vi "Manual User Input.vi"() -> (2 "XML":path, 3 "ZIP":path, 4 "Cancelled?":bool=TRUE)   [LabVIEW 2021]
panel:
  in  "Loc string":string="LabVIEW cannot reach the National Instruments Web server. You must synchronize with the Icon Library manually.\nClick the Help button for more information about resolving this error."
  in  "Help":bool
  in  "Icon library XML file":path
  in  "Icon library ZIP file":path
  out "Instructions":string
  in  "Cancel":bool
  in  "OK":bool
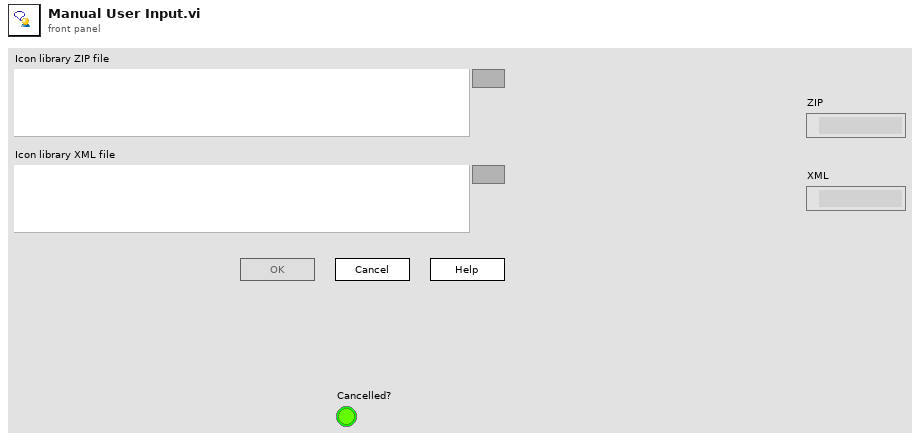
[diagram p1: front panel]
types:
  T1 = enum8{"Enabled", "Disabled", "Disabled and Grayed Out"}
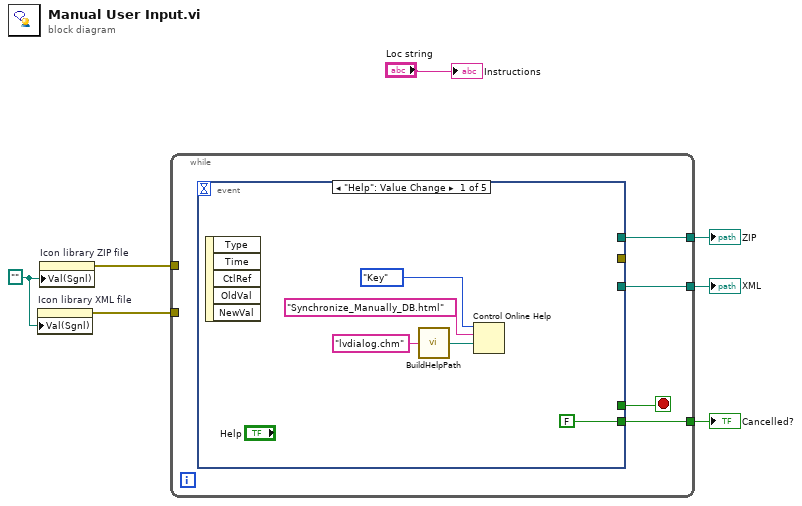
[diagram p0: block diagram]
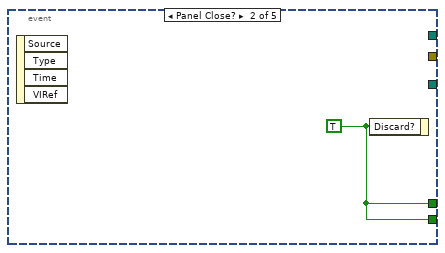
[diagram p2: hidden frame]
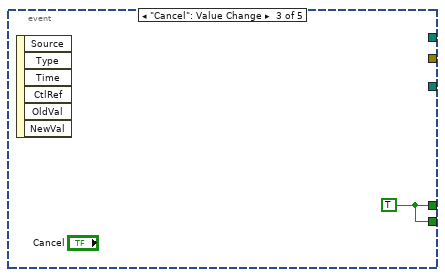
[diagram p3: hidden frame]
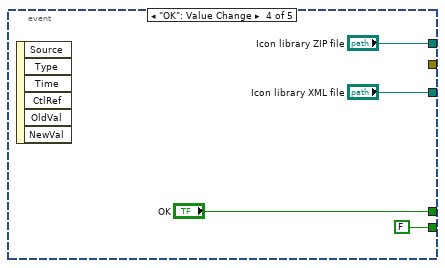
[diagram p4: hidden frame]
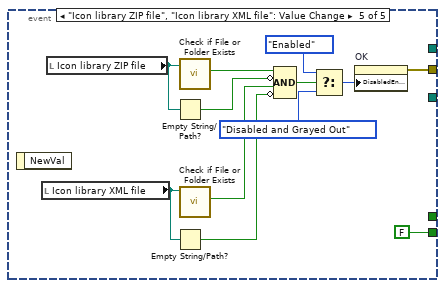
[diagram p5: hidden frame]
diagram:
  w5 = path ""
  n1 = property on="Icon library XML file" class="Path"("Val(Sgnl)"=w5) -> (error out=w2:errorcluster)  [unwired: 2 in, 1 out]
  n2 = property on="Icon library ZIP file" class="Path"("Val(Sgnl)"=w5) -> (error out=w3:errorcluster)  [unwired: 2 in, 1 out]
  n3 = while {
    tunnel: [w8] -> w7
    tunnel: [w11] -> w4
    tunnel: [w10] -> w6
    tunnel: w3 -> [_]
    tunnel: w2 -> [_]
    stop <- w9 stop-if-true
    n4 = event shown="[0] \"Help\": Value Change" {
      selector: _ -> [_ _ _ _ _]
      dyn-events: _ -> [_ _ _ _ _]
      timeout: _ -> [_ _ _ _ _]
      tunnel: [_ w17 w18 "OK" _] -> w9
      tunnel: [_ _ _ "Icon library ZIP file" _] -> w11
      tunnel: [_ _ _ "Icon library XML file" _] -> w10
      tunnel: [_ _ _ _ w24] -> _
      tunnel: [FALSE ("Discard?") w17 w18 FALSE ("Discard?") FALSE ("Discard?")] -> w8
      event "Help": Value Change {
        n5 = event-data() -> ()  [unwired: 1 in, 5 out]
        n6 = call <vilib>:"BuildHelpPath.vi"("Help File Name"="lvdialog.chm") -> ("Help File Path"=w14:path)
        n7 = Control Online Help(2:w14, 3:"Synchronize_Manually_DB.html" ("String to search for"), 4:enum16{"Contents", "Key", "Close"}."Key" ("Operation")) -> ()  [unwired: 1 in, 1 out]
      }
      event Panel Close? {
        w17 = TRUE ("Discard?")
        n8 = event-data() -> ()  [unwired: 1 in, 4 out]
        n9 = event-data("Discard?"=w17) -> ()  [unwired: 1 in, 1 out]
      }
      event "Cancel": Value Change {
        w18 = TRUE ("Discard?")
        n10 = event-data() -> ()  [unwired: 1 in, 6 out]
      }
      event "OK": Value Change {
        n11 = event-data() -> ()  [unwired: 1 in, 6 out]
      }
      event "Icon library ZIP file", "Icon library XML file": Value Change {
        n12 = event-data() -> ()  [unwired: 1 in, 1 out]
        n13 = local read "Icon library XML file"() -> (w33:path)
        n14 = local read "Icon library ZIP file"() -> (w34:path)
        n15 = Empty String/Path?(string/path=w34) -> (empty?=w31:bool)
        n16 = Empty String/Path?(string/path=w33) -> (empty?=w29:bool)
        n17 = call <vilib>:"Check if File or Folder Exists.vi"("path"=w34) -> ("file or folder exists?"=w32:bool)  [unwired: 8 in, 2 out]
        n18 = call <vilib>:"Check if File or Folder Exists.vi"("path"=w33) -> ("file or folder exists?"=w30:bool)  [unwired: 8 in, 2 out]
        n19 = Compound Arithmetic op=AND(w32, invert w31, w30, invert w29) -> (w28:bool)
        n20 = Select(t=T1."Enabled" ("Disabled"), s=w28, f=T1."Disabled and Grayed Out" ("Disabled")) -> (s? t:f=w27:T1)
        n21 = property on="OK" class="Bool"("DisabledEnum"=w27) -> (error out=w24:errorcluster)  [unwired: 2 in, 1 out]
      }
    }
  }
  "Cancelled?" <- w7
  "ZIP" <- w4
  "XML" <- w6
  "Instructions" <- "Loc string"
